vi "GE5565 Read (U32) Cluster mod.vi"(7 "Address Space":T1=1 items=["VXI/VME A16"=1, "VXI/VME A24"=2, "VXI/VME A32"=3, "VXI/VME A64"=4, "PXI Memory Allocations"=9, "PXI Configuration"=10, "PXI BAR0"=11, "PXI BAR1"=12, "PXI BAR2"=13, "PXI BAR3"=14, "PXI BAR4"=15, "PXI BAR5"=16], 8 "error in (no error)":errorcluster, 10 "offset (0)":u32, 11 "VMIC reference in":T2) -> (0 "error out":errorcluster, 2 "Data":u32, 3 "VMIC reference out":T2)   [LabVIEW 2020, in "RefMem DMA Engine.lvlib"]
uses:
  RefMem DMA Engine.lvlib
  <vilib>/Instr/_visa.llb/VISA Register Access Address Space.ctl
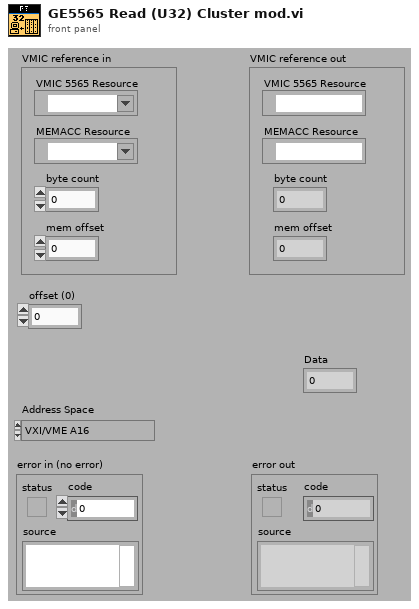
[diagram p1: front panel]
types:
  T1 = typedef "VISA Register Access Address Space.ctl" = u16
  T2 = cluster{"VMIC 5565 Resource":refnum<visa-resource-name>, "MEMACC Resource":refnum<visa-resource-name>, "byte count":u32, "mem offset":u32}
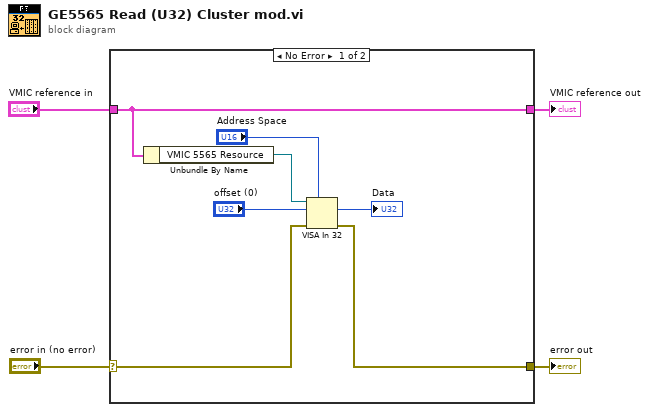
[diagram p0: block diagram]
diagram:
  n1 = case shown="No Error" "error in (no error)" {
    selector: "error in (no error)" -> [w11 w12]
    tunnel: "VMIC reference in" -> [w9 w13]
    tunnel: [w9 w13] -> w1
    tunnel: [w10 w12] -> w3
    frame No Error {
      n2 = Unbundle By Name(w9) -> ("VMIC 5565 Resource"=w7:refnum<visa-resource-name>)
      n3 = VISA In 32(7:"Address Space", 8:w11, 10:"offset (0)", 11:w7) -> (0:w10:errorcluster, 2:→"Data":u32)  [unwired: 1 out]
    }
    frame Error {
    }
  }
  "error out" <- w3
  "VMIC reference out" <- w1
